vi "Get CIPC Channel.vi"(8 "error in (no error)":errorcluster, 11 "CIF_CIPC_Chn in":refnum<class "CIF_CIPC_Chn.lvclass">) -> (0 "error out":errorcluster, 2 "CIPC Channel":u64, 3 "CIF_CIPC_Chn out":refnum<class "CIF_CIPC_Chn.lvclass">)   [LabVIEW 2021, in "CIF_CIPC_Chn.lvclass"]
uses:
  CIF_CIPC_Chn.lvclass
  CIF_CIPC_Chn.lvclass/CIF_CIPC_Chn.ctl
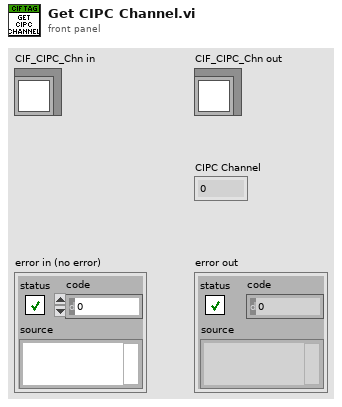
[diagram p1: front panel]
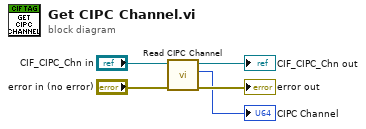
[diagram p0: block diagram]
diagram:
  n1 = call "Read CIPC Channel.vi"("error in (no error)"="error in (no error)", "CIFTag in"="CIF_CIPC_Chn in") -> ("error out"=→"error out":errorcluster, "CIF Channel"=→"CIPC Channel":u64, "CIFTag out"=→"CIF_CIPC_Chn out":refnum<class "CIF_CIPC_Chn.lvclass">)  [unwired: 7 in]
